vi "Analog Output - 1 Channel - Continuous Sampling.vi"() -> ()   [LabVIEW 2019]
uses:
  <vilib>/myRIO/Instrument Drivers/Onboard IO/AO Continuous/typedefs/AO Continuous Reference.ctl
  <vilib>/myRIO/Common/Instrument Driver Framework/Utilities/typedefs/myRIO Generic Hardware Reference.ctl
  <vilib>/myRIO/Common/Instrument Driver Framework/Utilities/typedefs/Hardware Version Enum.ctl
  <vilib>/myRIO/Common/Instrument Driver Framework/Utilities/typedefs/myRIO v1.0 Reference.ctl
  <vilib>/myRIO/Common/Instrument Driver Framework/Utilities/typedefs/Generic FPGA Reference.ctl
  <vilib>/myRIO/Common/Instrument Driver Framework/ELVIS III v1.0/AO Continuous/typedefs/AO Continuous Channels List.ctl
  <vilib>/myRIO/Common/Instrument Driver Framework/ELVIS III v1.0/AO Continuous/typedefs/ELVIS III v1.0 AO Continuous Channels Enum.ctl
  <vilib>/myRIO/Common/Instrument Driver Framework/ELVIS III v1.0/AO Continuous/typedefs/AO Continuous Channel Info.ctl
  <vilib>/userdefined/High Color/nirio_resource_hc.ctl
  <vilib>/myRIO/Common/Instrument Driver Framework/ELVIS III v1.0/AO Continuous/vis/ELVIS III v1.1 Open AO (Continuous).vi
  <vilib>/myRIO/Common/Instrument Driver Framework/Utilities/vis/Validate Channels.vi
  <vilib>/myRIO/Common/Instrument Driver Framework/ELVIS III v1.0/AO Continuous/vis/ELVIS III v1.0 Reserve AO Continuous.vi
  <vilib>/myRIO/Common/Instrument Driver Framework/ELVIS III v1.0/AO Continuous/vis/ELVIS III v1.1 Close AO Continuous.vi
  <vilib>/myRIO/Common/Instrument Driver Framework/myRIO v1.0/UART/vis/myRIO v1.0 Close UART.vi
  <vilib>/myRIO/Common/Instrument Driver Framework/ELVIS III v1.0/AO Continuous/vis/ELVIS III v1.0 Build MUX Configuration AO Continuous.vi
  <vilib>/myRIO/Common/Instrument Driver Framework/ELVIS III v1.0/AO Continuous/vis/ELVIS III v1.0 Unreserve AO Continuous.vi
  <vilib>/Utility/VariantDataType/GetNumericInfo.vi
  <vilib>/Utility/error.llb/Error Cluster From Error Code.vi
  <vilib>/myRIO/Common/Instrument Driver Framework/ELVIS III v1.0/ELVIS III v1.1 Open.vi
  <vilib>/myRIO/Common/Instrument Driver Framework/ELVIS III v1.0/Resource Manager/vis/ELVIS III v1.0 Reserve Channel List.vi
  <vilib>/myRIO/Common/Instrument Driver Framework/ELVIS III v1.0/Resource Manager/vis/ELVIS III v1.0 Configure DMAs.vi
  <vilib>/myRIO/Common/Instrument Driver Framework/myRIO v1.0/myRIO v1.0 Close.vi
  <vilib>/myRIO/Common/Instrument Driver Framework/ELVIS III v1.0/AO Continuous/vis/ELVIS III v1.1 Stop AO Continuous.vi
  <vilib>/myRIO/Common/Instrument Driver Framework/ELVIS III v1.0/AO Continuous/vis/ELVIS III v1.1 Start AO Continuous.vi
  <vilib>/myRIO/Common/Instrument Driver Framework/ELVIS III v1.0/AO Continuous/vis/ELVIS III v1.0 AO Continuous Write.vi
  <vilib>/myRIO/Common/Instrument Driver Framework/ELVIS III v1.0/Resource Manager/vis/ELVIS III v1.0 Unreserve Channel List.vi
  <vilib>/myRIO/Common/Instrument Driver Framework/Utilities/vis/FPGA Ref Manager.vi
  <vilib>/myRIO/Common/Instrument Driver Framework/ELVIS III v1.0/ELVIS III v1.0 Reset FPGA.vi
  <vilib>/myRIO/Common/Instrument Driver Framework/myRIO v1.0/IRQ/vis/myRIO v1.0 IRQ Info FGV.vi
  <vilib>/myRIO/Common/Instrument Driver Framework/myRIO v1.0/IRQ/vis/myRIO v1.0 Timer IRQ Info FGV.vi
  <vilib>/myRIO/Common/Instrument Driver Framework/myRIO v1.0/IRQ/vis/myRIO v1.0 ISR Agent.vi
  <vilib>/myRIO/Instrument Drivers/Utilities/vis/Reset Index.vi
  <vilib>/myRIO/Common/Instrument Driver Framework/myRIO v1.0/Resource Manager/vis/myRIO v1.0 Block Write Resource Manager.vi
  <vilib>/myRIO/Instrument Drivers/Onboard IO/AO Continuous/vis/myRIO AO Continuous Open.xnode
  <vilib>/myRIO/Instrument Drivers/Utilities/Utilities.lvlib
  <vilib>/myRIO/Instrument Drivers/Onboard IO/AO Continuous/AO Continuous.lvlib
panel:
  in  "Stop":bool
  in  "Amplitude (V)":dbl=5.0 min=-10.0 max=10.0 step=0.1 format="%#_13g"
  in  "Frequency (Hz)":dbl=10.0 format="%#_13g"
  in  "Generate Waveform":bool
  # "ELVIS III Control IO"
  # "模拟输入单通道"
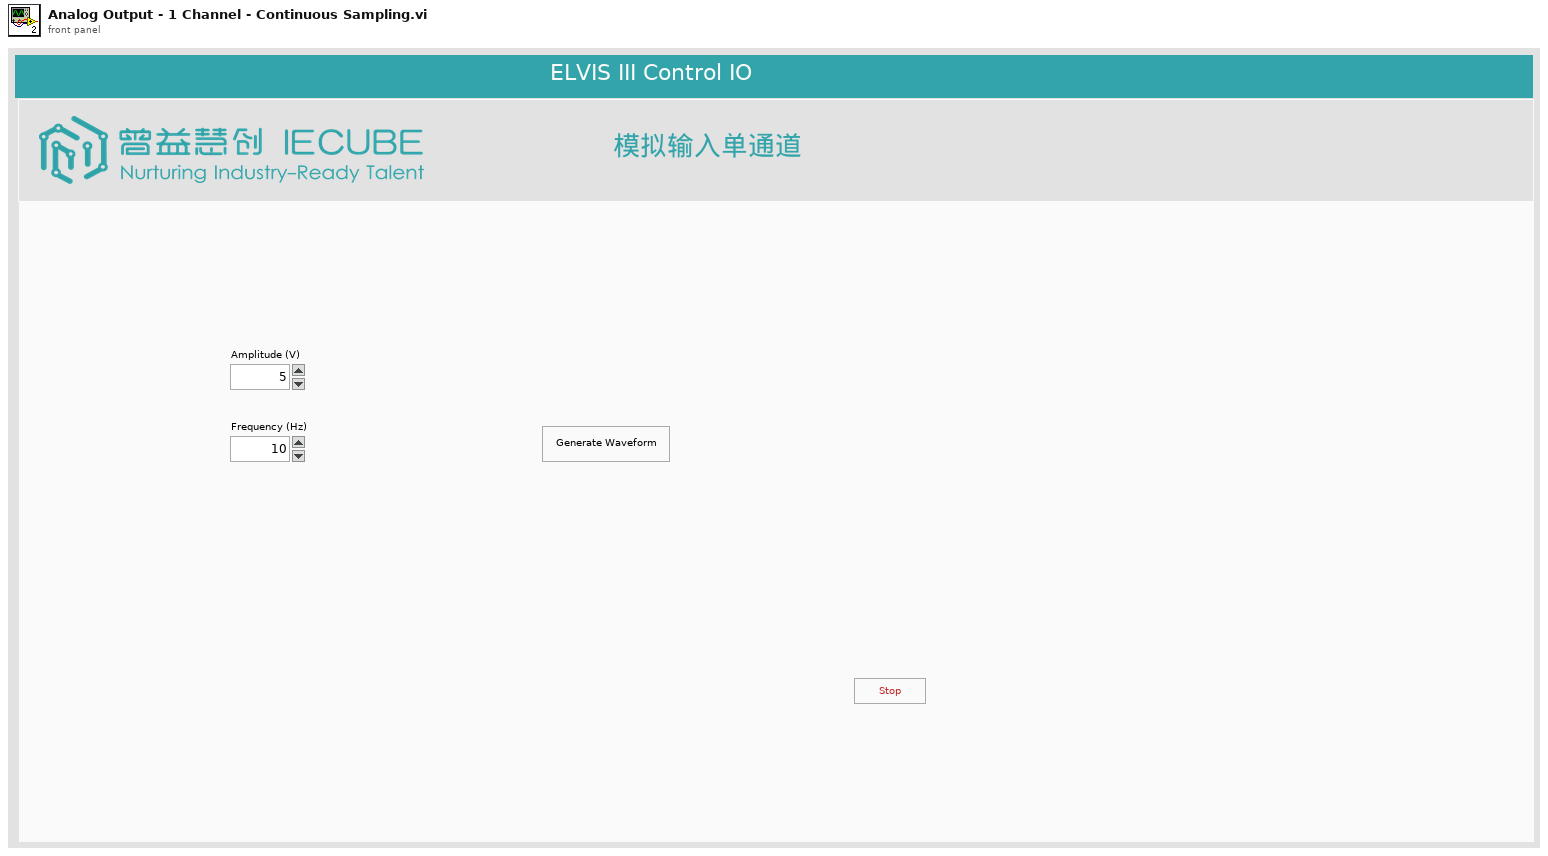
[diagram p1: front panel]
types:
  T1 = typedef "nirio_resource_hc.ctl" = tag
  T2 = typedef "Hardware Version Enum.ctl" = enum16{"Unknown", "myRIO-1900", "myRIO-1950", "roboRIO", "NI ELVIS RIO CM", "ELVIS III"}
  T3 = typedef "AO Continuous.lvlib/AO Continuous Reference.ctl" = cluster{"myRIO Reference":T4, "AO (Continuous) Channels List":T7, "Channel Info":T9}
  T4 = typedef "myRIO Generic Hardware Reference.ctl" = cluster{"myRIO Model":T2, "myRIO Hardware Reference":T5}
  T5 = typedef "myRIO v1.0 Reference.ctl" = cluster{"Generic FPGA Reference":T6, "Allow multiple opens":bool}
  T6 = typedef "Generic FPGA Reference.ctl" = refnum<k20>
  T7 = typedef "AO Continuous Channels List.ctl" = T8[]
  T8 = typedef "ELVIS III v1.0 AO Continuous Channels Enum.ctl" = enum16{"Not Connected", "A/AO0 (Continuous)", "A/AO1 (Continuous)", "B/AO0 (Continuous)", "B/AO1 (Continuous)"}
  T9 = typedef "AO Continuous Channel Info.ctl" = cluster{"Channel Bitmask":u8[], "Channel Index":i32[], "Channel Number":u8}
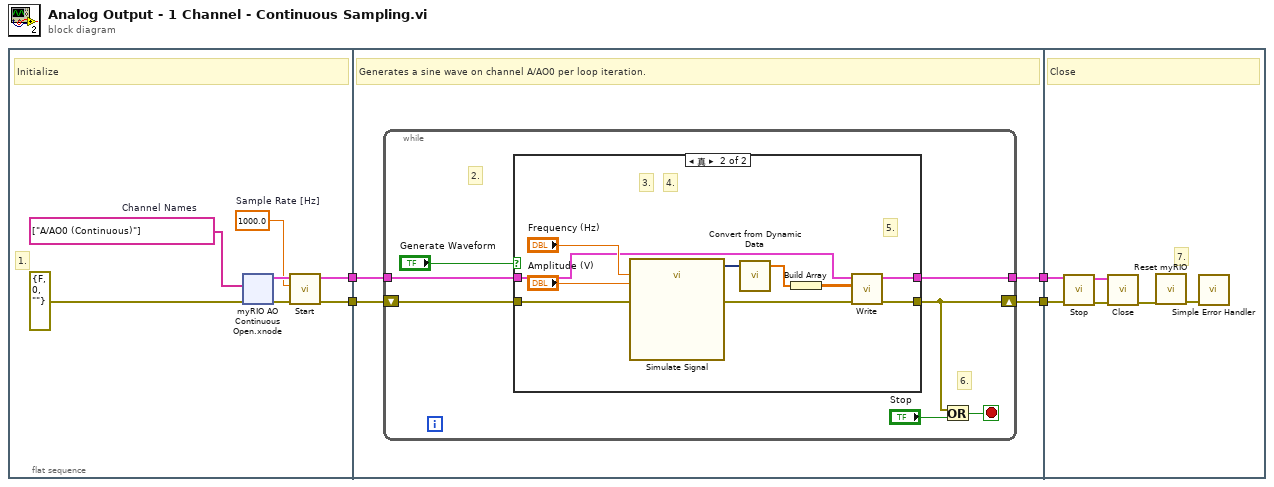
[diagram p0: block diagram]
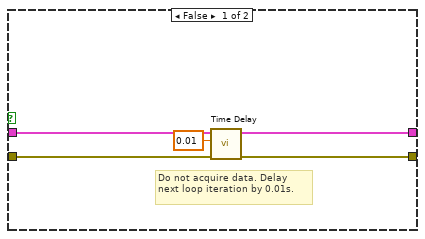
[diagram p2: hidden frame]
diagram:
  n1 = flat-sequence {
    tunnel: [w8] -> w4
    tunnel: [w7] -> w3
    tunnel: [w32] -> w2
    tunnel: w4 -> [w31]
    tunnel: [w30] -> w1
    tunnel: w3 -> [w29]
    tunnel: w2 -> [w56]
    tunnel: w1 -> [w55]
    frame #0 {
      w6 = tag[] ["A/AO0 (Continuous)"]  # Channel Names
      w5 = 1000.0  # Sample Rate [Hz]
      # "1."
      # "Initialize"
      n2 = xnode "myRIO AO Continuous Open.xnode"("error in (no error)"=errorcluster {"status"=FALSE, "code"=0, "source"=""} ("Error In"), "Channel Names"=w6) -> ("error out"=w11:errorcluster, "AO (Continuous) Ref Out"=w10:T3)
      n3 = call <vilib>:"Start.vi"("error in (no error)"=w11, "Sample Rate"=w5, "AO (Continuous) Ref In"=w10) -> ("error out"=w8:errorcluster, "AO (Continuous) Ref Out"=w7:T3)  [unwired: 7 in]
    }
    frame #1 {
      # "Generates a sine wave on channel A/AO0 per loop iteration."
      n4 = while {
        shift-right: [w38] -> w32
        shift-left: w31 -> [w37]
        tunnel: [w34] -> w30
        tunnel: w29 -> [w33]
        stop <- w39 stop-if-true
        # "6."
        # "2."
        n5 = case shown="真" "Generate Waveform" {
          tunnel: [w42 w48] -> w38
          tunnel: w37 -> [w41 w53]
          tunnel: [w40 w45] -> w34
          tunnel: w33 -> [w40 w46]
          frame False {
            # "Do not acquire data. Delay next loop iteration by 0.01s."
            n6 = call "Time Delay"("error in (no error)"=w41, "Delay Time (s)"=0.01) -> ("error out"=w42:errorcluster)  [unwired: 9 in]
          }
          frame True {
            # "5."
            # "4."
            # "3."
            n7 = call "Simulate Signal"("Frequency"="Frequency (Hz)", "Amplitude"="Amplitude (V)", "error in (no error)"=w53) -> ("Sine"=w50:dynamicdata, "error out"=w47:errorcluster)  [unwired: 11 in]
            n8 = call "Convert from Dynamic Data"("Dynamic Data Type"=w50) -> ("Array"=w49:dbl[])  [unwired: 3 in]
            n9 = Build Array(w49) -> (w44:dbl[][])
            n10 = call <vilib>:"Write.vi"("error in (no error)"=w47, "Data To Write"=w44, "AO (Continuous) Ref In"=w46) -> ("error out"=w48:errorcluster, "AO (Continuous) Ref Out"=w45:T3)  [unwired: 7 in]
          }
        }
        n11 = Or(x=w38, y="Stop") -> (x .or. y?=w39:bool)
      }
    }
    frame #2 {
      # "7."
      # "Close"
      n12 = call <vilib>:"Stop.vi"("error in (no error)"=w56, "AO (Continuous) Ref In"=w55) -> ("error out"=w57:errorcluster, "AO (Continuous) Ref Out"=w58:T3)  [unwired: 8 in]
      n13 = call <vilib>:"Close.vi"("error in (no error)"=w57, "AO (Continuous) Ref In"=w58) -> ("error out"=w54:errorcluster)  [unwired: 9 in]
      n14 = call <vilib>:"Reset myRIO.vi"("error in (no error)"=w54) -> ("error out"=w59:errorcluster)  [unwired: 10 in]
      n15 = call <vilib>:"Simple Error Handler.vi"("error in (no error)"=w59) -> ()  [unwired: 4 in, 5 out]
    }
  }
